vi "ziModUnSubscribe.vi"(8 "Error In":errorcluster, 10 "Path (\"/\")":string="/", 11 "ModHandle In":T1 {"ModHandle" format="0x%08x"; "Conn" format="0x%08x"}) -> (0 "Error Out":errorcluster, 3 "ModHandle Out":T1 {"ModHandle" format="0x%08x"; "Conn" format="0x%08x"})   [LabVIEW 2015, in "Zurich Instruments LabOne.lvlib"]
doc: "This vi is the complement to ziModSubscribe.vi and unsubsribes from a node."
uses:
  Zurich Instruments LabOne.lvlib
  Zurich Instruments/LabOne/API/LabVIEW/Zurich Instruments LabOne/Private/ziLV64.framework
  ziTypeModHandle.ctl
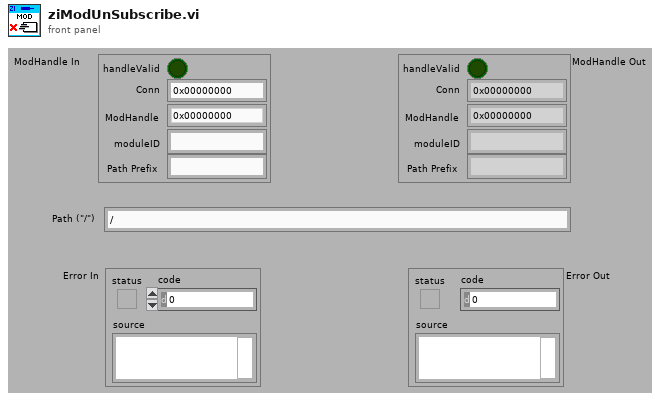
[diagram p1: front panel]
types:
  T1 = typedef "Zurich Instruments LabOne.lvlib/ziTypeModHandle.ctl" = cluster{"handleValid":bool, "Conn":u64, "ModHandle":u64, "moduleID":string, "Path Prefix":string}
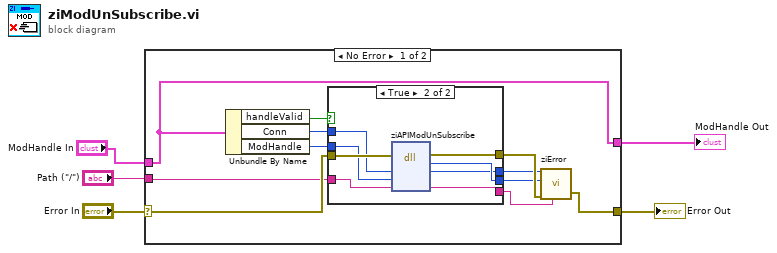
[diagram p0: block diagram]
diagram:
  n1 = case shown="No Error" "Error In" {
    selector: "Error In" -> [w14 w28]
    tunnel: [w8 w28] -> w5
    tunnel: [w11 w27] -> w1
    tunnel: "Path (\"/\")" -> [w13 _]
    tunnel: "ModHandle In" -> [w11 w27]
    frame No Error {
      n2 = Unbundle By Name(w11) -> ("handleValid"=w16:bool, "Conn"=w15:u64, "ModHandle"=w12:u64)
      n3 = case shown="True" w16 {
        tunnel: w14 -> [w18 w26]
        tunnel: w15 -> [w17 w25]
        tunnel: [w18 w24] -> w10
        tunnel: w13 -> [_ w23]
        tunnel: w12 -> [_ w22]
        tunnel: [_ w21] -> w9
        tunnel: [_ w20] -> w7
        tunnel: [w17 w19] -> w6
        frame False {
        }
        frame True {
          n4 = dll-call lib="Users/arkady/Desktop/ado/github/resonant_ultrasound_arxiv/maglab ultrasound -- arkady --arxiv/Zurich Instruments/LabOne/API/LabVIEW/Zurich Instruments LabOne/Private/ziLV*.*" fn="ziAPIModUnSubscribe" label="ziAPIUnSubscribe"(error in=w26, "Conn"=w25, "ModHandle"=w22, "Path"=w23) -> (error out=w24:errorcluster, "return type"=w21:u32, "Conn"=w19:u64, "Path"=w20:string)  [unwired: 3 in, 1 out]
        }
      }
      n5 = call "ziError.vi"("Conn"=w6, "ziErrorCode"=w9, "Error In"=w10, "Annotation"=w7) -> ("Error Out"=w8:errorcluster)  [unwired: 1 in, 1 out]
    }
    frame Error {
    }
  }
  "Error Out" <- w5
  "ModHandle Out" <- w1
